vi "Delete Item.vi"(6 "Data":variant, 8 "error in (no error)":errorcluster, 9 "Tag string":string, 10 "Tag":refnum<class "Tree Tag Class.lvclass">, 11 "Tree_LVOOP in":refnum<class "Tree Class.lvclass">) -> (0 "error out":errorcluster, 2 "Deleted Tag":refnum<class "Tree Tag Class.lvclass">, 3 "Tree_LVOOP out":refnum<class "Tree Class.lvclass">)   [LabVIEW 2012, in "Tree Tools.lvlib" / "Tree Class.lvclass"]
uses:
  Tree Class.lvclass
  Tree Tag Class/Tree Tag Class.lvclass
  Tree Class.lvclass/Tree Class.ctl
panel:
  out "Array 3":string[](array[string])
  out "Array 2":i32[](array[numeric])
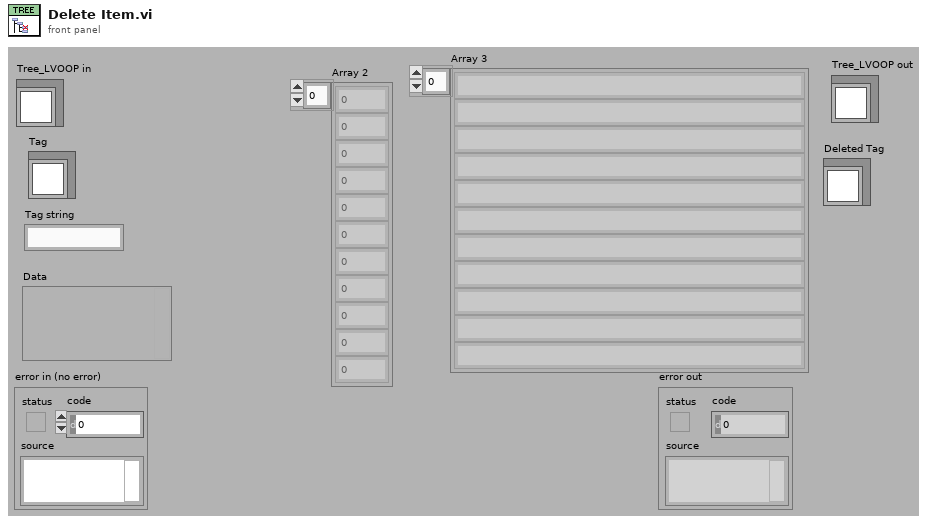
[diagram p1: front panel]
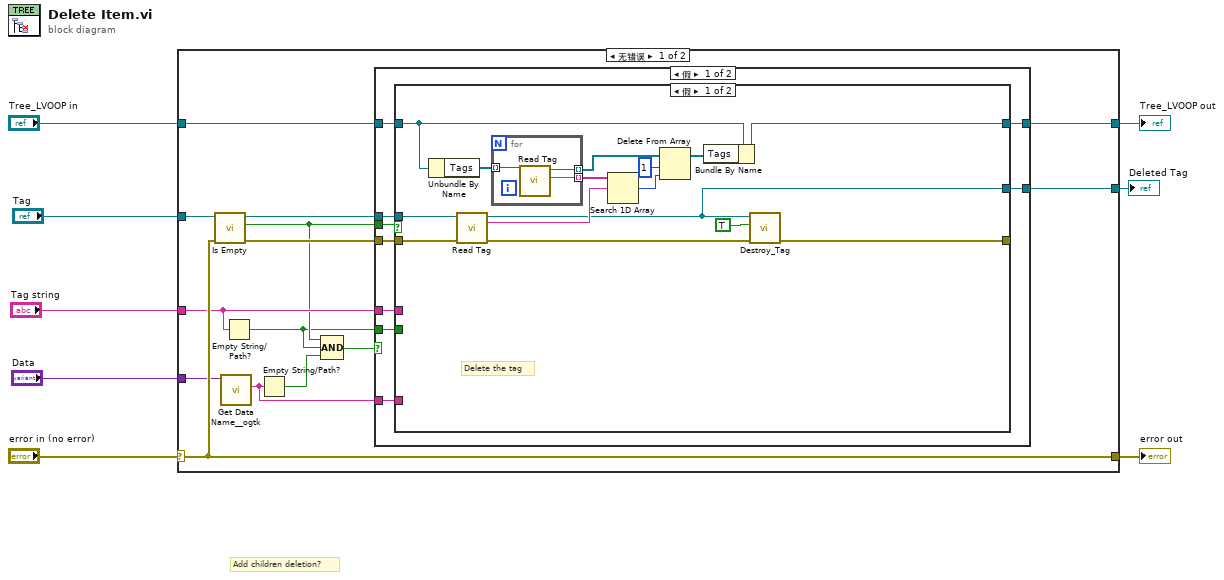
[diagram p0: block diagram]
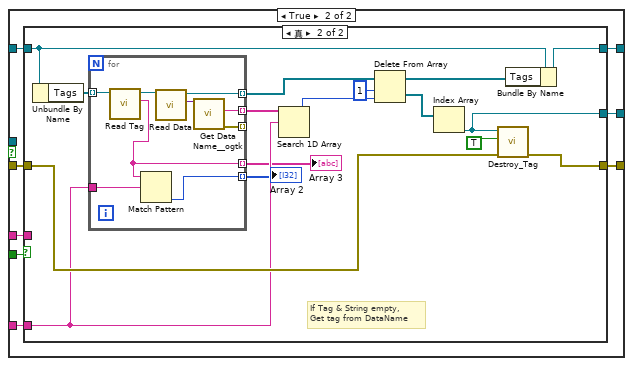
[diagram p2: hidden frame]
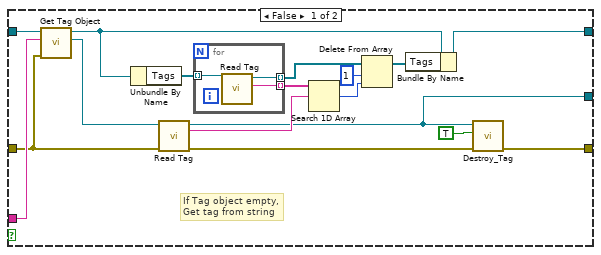
[diagram p3: hidden frame]
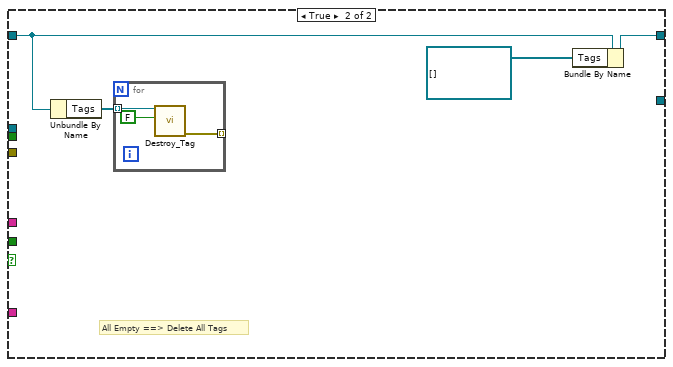
[diagram p4: hidden frame]
diagram:
  # "Add children deletion?"
  n1 = case shown="无错误" "error in (no error)" {
    selector: "error in (no error)" -> [w17 w111]
    tunnel: [w17 w111] -> w7
    tunnel: [w20 w110] -> w5
    tunnel: "Tree_LVOOP in" -> [w21 w110]
    tunnel: "Tag" -> [w22 _]
    tunnel: "Tag string" -> [w15 _]
    tunnel: "Data" -> [w16 _]
    tunnel: [w9 _] -> w1
    frame No Error {
      n2 = call-dynamic "Is Empty.vi"("error in (no error)"=w17, "Tag_LVOOP in"=w22) -> ("error out"=w18:errorcluster, "Empty"=w13:bool, "Tag_LVOOP out"=w19:refnum<class "Tree Tag Class.lvclass">)  [unwired: 7 in]
      n3 = call <userlib>:"Get Data Name__ogtk.vi"("Data"=w16) -> ("Data Name"=w10:string)  [unwired: 1 in, 9 out]
      n4 = Empty String/Path?(string/path=w15) -> (empty?=w11:bool)
      n5 = Empty String/Path?(string/path=w10) -> (empty?=w14:bool)
      n6 = Compound Arithmetic op=AND(w13, w11, w14) -> (w12:bool)
      n7 = case shown="假" w12 {
        tunnel: w21 -> [w31 w106]
        tunnel: [w30 w105] -> w20
        tunnel: w19 -> [w29 _]
        tunnel: w18 -> [w28 _]
        tunnel: w15 -> [w27 _]
        tunnel: w13 -> [w26 _]
        tunnel: w11 -> [w25 _]
        tunnel: w10 -> [w24 _]
        tunnel: [w23 _] -> w9
        frame False {
          n8 = case shown="假" w26 {
            tunnel: w31 -> [w46 w57]
            tunnel: [w45 w55] -> w30
            tunnel: w27 -> [_ w56]
            tunnel: w29 -> [w41 _]
            tunnel: w28 -> [w40 w53]
            tunnel: [w43 w54] -> _
            tunnel: w25 -> [_ w52]
            tunnel: w24 -> [_ w51]
            tunnel: [w32 w50] -> w23
            frame False {
              # "Delete the tag"
              n9 = Unbundle By Name(w46) -> ("Tags"=w39:refnum<class "Tree Tag Class.lvclass">[])
              n10 = call-dynamic "Read Tag.vi"("error in (no error)"=w40, "Tag_LVOOP.lvclass in"=w41) -> ("error out"=w42:errorcluster, "Tag"=w37:string, "Tag_LVOOP.lvclass out"=w32:refnum<class "Tree Tag Class.lvclass">)  [unwired: 7 in]
              n11 = for {
                tunnel: w39 -> [w49] mode=indexing
                tunnel: [w48] -> w38 mode=indexing
                tunnel: [w47] -> w36 mode=indexing
                n12 = call-dynamic "Read Tag.vi"("Tag_LVOOP.lvclass in"=w49) -> ("Tag"=w48:string, "Tag_LVOOP.lvclass out"=w47:refnum<class "Tree Tag Class.lvclass">)  [unwired: 8 in, 1 out]
              }
              n13 = Search 1D Array(1D array=w38, element=w37) -> (index of element=w33:i32)  [unwired: 1 out]
              n14 = Delete From Array(array=w36, length=1, index=w33) -> (array with subset deleted=w35:refnum<class "Tree Tag Class.lvclass">[])  [unwired: 1 out]
              n15 = Bundle By Name(cluster=w46, "Tags"=w35) -> (w45:refnum<class "Tree Class.lvclass">)
              n16 = call-dynamic "Destroy_Tag.vi"("error in (no error)"=w42, "Delete Children? (F)"=TRUE, "Tag_LVOOP in"=w32) -> ("error out"=w43:errorcluster)  [unwired: 8 in]
            }
            frame True {
              n17 = case shown="真" w52 {
                tunnel: w57 -> [w74 w85]
                tunnel: w56 -> [w73 _]
                tunnel: [w62 w84] -> w55
                tunnel: [w61 w83] -> w54
                tunnel: w53 -> [w60 w81]
                tunnel: w51 -> [_ w80]
                tunnel: [w58 w82] -> w50
                frame False {
                  # "If Tag object empty,\nGet tag from string"
                  n18 = call-dynamic "Get Tag Object.vi"("error in (no error)"=w60, "Tag (string)"=w73, "Tree_LVOOP in"=w74) -> ("Tag"=w59:refnum<class "Tree Tag Class.lvclass">, "Tree_LVOOP out"=w63:refnum<class "Tree Class.lvclass">)  [unwired: 1 in, 6 out]
                  n19 = Unbundle By Name(w63) -> ("Tags"=w70:refnum<class "Tree Tag Class.lvclass">[])
                  n20 = call-dynamic "Read Tag.vi"("error in (no error)"=w60, "Tag_LVOOP.lvclass in"=w59) -> ("error out"=w71:errorcluster, "Tag"=w68:string, "Tag_LVOOP.lvclass out"=w58:refnum<class "Tree Tag Class.lvclass">)  [unwired: 7 in]
                  n21 = for {
                    tunnel: w70 -> [w77] mode=indexing
                    tunnel: [w76] -> w69 mode=indexing
                    tunnel: [w75] -> w67 mode=indexing
                    n22 = call-dynamic "Read Tag.vi"("Tag_LVOOP.lvclass in"=w77) -> ("Tag"=w76:string, "Tag_LVOOP.lvclass out"=w75:refnum<class "Tree Tag Class.lvclass">)  [unwired: 8 in, 1 out]
                  }
                  n23 = Search 1D Array(1D array=w69, element=w68) -> (index of element=w64:i32)  [unwired: 1 out]
                  n24 = Delete From Array(array=w67, length=1, index=w64) -> (array with subset deleted=w66:refnum<class "Tree Tag Class.lvclass">[])  [unwired: 1 out]
                  n25 = Bundle By Name(cluster=w63, "Tags"=w66) -> (w62:refnum<class "Tree Class.lvclass">)
                  n26 = call-dynamic "Destroy_Tag.vi"("error in (no error)"=w71, "Delete Children? (F)"=TRUE, "Tag_LVOOP in"=w58) -> ("error out"=w61:errorcluster)  [unwired: 8 in]
                }
                frame True {
                  # "If Tag & String empty,\nGet tag from DataName"
                  n27 = Unbundle By Name(w85) -> ("Tags"=w93:refnum<class "Tree Tag Class.lvclass">[])
                  n28 = for {
                    tunnel: w93 -> [w97] mode=indexing
                    tunnel: [w95] -> w92 mode=indexing
                    tunnel: [w101] -> w88 mode=indexing
                    tunnel: [w100] -> _ mode=indexing
                    tunnel: w80 -> [w99]
                    tunnel: [w98] -> w79 mode=indexing
                    tunnel: [w94] -> w78 mode=indexing
                    n29 = call-dynamic "Read Tag.vi"("Tag_LVOOP.lvclass in"=w97) -> ("Tag"=w94:string, "Tag_LVOOP.lvclass out"=w96:refnum<class "Tree Tag Class.lvclass">)  [unwired: 8 in, 1 out]
                    n30 = Match Pattern(string=w94, regular expression=w99) -> (offset past match=w98:i32)  [unwired: 4 out]
                    n31 = call-dynamic "Read Data.vi"("Tag_LVOOP.lvclass in"=w96) -> ("Data"=w102:variant, "Tag_LVOOP.lvclass out"=w101:refnum<class "Tree Tag Class.lvclass">)  [unwired: 8 in, 1 out]
                    n32 = call <userlib>:"Get Data Name__ogtk.vi"("Data"=w102) -> ("error out"=w100:errorcluster, "Data Name"=w95:string)  [unwired: 1 in, 8 out]
                  }
                  "Array 2" <- w79
                  "Array 3" <- w78
                  n33 = Search 1D Array(1D array=w92, element=w80) -> (index of element=w87:i32)  [unwired: 1 out]
                  n34 = Delete From Array(array=w88, length=1, index=w87) -> (deleted portion=w86:refnum<class "Tree Tag Class.lvclass">[], array with subset deleted=w90:refnum<class "Tree Tag Class.lvclass">[])
                  n35 = Index Array(array=w86) -> (element=w82:refnum<class "Tree Tag Class.lvclass">)  [unwired: 1 in]
                  n36 = call-dynamic "Destroy_Tag.vi"("error in (no error)"=w81, "Delete Children? (F)"=TRUE, "Tag_LVOOP in"=w82) -> ("error out"=w83:errorcluster)  [unwired: 8 in]
                  n37 = Bundle By Name(cluster=w85, "Tags"=w90) -> (w84:refnum<class "Tree Class.lvclass">)
                }
              }
            }
          }
        }
        frame True {
          # "All Empty ==> Delete All Tags"
          n38 = Unbundle By Name(w106) -> ("Tags"=w103:refnum<class "Tree Tag Class.lvclass">[])
          n39 = for {
            tunnel: w103 -> [w109] mode=indexing
            tunnel: [w107] -> _ mode=indexing
            n40 = call-dynamic "Destroy_Tag.vi"("Delete Children? (F)"=FALSE, "Tag_LVOOP in"=w109) -> ("error out"=w107:errorcluster)  [unwired: 9 in]
          }
          n41 = Bundle By Name(cluster=w106, "Tags"=refnum<class "Tree Tag Class.lvclass">[] []) -> (w105:refnum<class "Tree Class.lvclass">)
        }
      }
    }
    frame Error {
    }
  }
  "error out" <- w7
  "Tree_LVOOP out" <- w5
  "Deleted Tag" <- w1
